vi "Read Line.vi"(8 "error in (no error)":errorcluster, 11 "DigitalEffectorHardware in":refnum<class "TTLControlledDevice.lvclass">) -> (0 "error out":errorcluster, 2 "Line":string, 3 "DigitalEffectorHardware out":refnum<class "TTLControlledDevice.lvclass">)   [LabVIEW 2020, in "TTLControlledDevice.lvclass"]
uses:
  TTLControlledDevice.lvclass
  TTLControlledDevice.lvclass/TTLControlledDevice.ctl
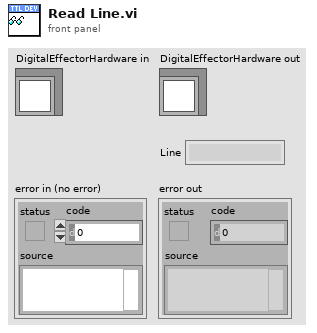
[diagram p1: front panel]
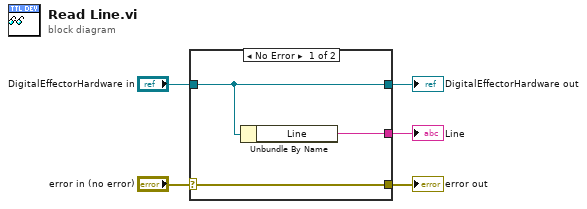
[diagram p0: block diagram]
diagram:
  n1 = case shown="No Error" "error in (no error)" {
    selector: "error in (no error)" -> [w8 w9]
    tunnel: [w8 w9] -> w4
    tunnel: [w7 w10] -> w2
    tunnel: "DigitalEffectorHardware in" -> [w7 w10]
    tunnel: [w6 _] -> w1
    frame No Error {
      n2 = Unbundle By Name(w7) -> ("Line"=w6:string)
    }
    frame Error {
    }
  }
  "error out" <- w4
  "DigitalEffectorHardware out" <- w2
  "Line" <- w1
